vi "DataSync.vi"(8 "method":i32(ring)=1 caption="메소드" items=["최근접", "선형", "스플라인", "3차 에르미트", "라그랑지"], 9 "samples":i32=3000 caption="샘플", 10 "Y":dbl[](array[numeric]) format="%_6g", 11 "X":dbl[](array[numeric]) format="%_6g") -> (1 "yi":dbl[](array[numeric]) format="%_6g", 2 "xi used":dbl[](array[numeric]) caption="사용된 xi" format="%_6g", 3 "출력 웨이브폼":waveform(dbl))   [LabVIEW 2013]
uses:
  <vilib>/Analysis/1siggen.llb/Ramp Pattern by Samples.vi
  <vilib>/Analysis/NI_AALBase.lvlib
  <vilib>/gmath/NI_Gmath.lvlib
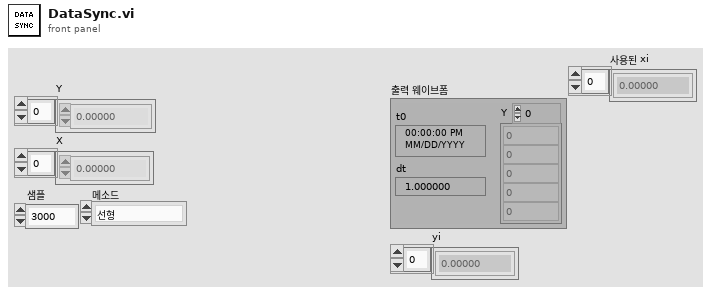
[diagram p1: front panel]
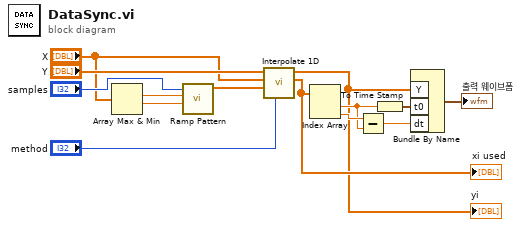
[diagram p0: block diagram]
diagram:
  n1 = Array Max & Min(array="X") -> (max value=w7:dbl, min value=w6:dbl)  [unwired: 2 out]
  n2 = call-poly <vilib>:"Ramp Pattern.vi"("start"=w6, "end"=w7, "samples"="samples") -> ("Ramp Pattern"=w14:dbl[])  [unwired: 7 in, 1 out]
  n3 = call <vilib>:"Interpolate 1D.vi"("method"="method", "xi"=w14, "X"="X", "Y"="Y") -> ("xi used"=w13:dbl[], "yi"=w8:dbl[])  [unwired: 5 in, 1 out]
  "yi" <- w8
  "xi used" <- w13
  n4 = Index Array(array=w13) -> (element #1=w10:dbl, element #2=w11:dbl)  [unwired: 2 in]
  n5 = Subtract(x=w11, y=w10) -> (x-y=w9:dbl)
  n6 = To Time Stamp(1:w10) -> (0:w12:timestamp)
  n7 = Bundle By Name("Y"=w8, "t0"=w12, "dt"=w9) -> (→"출력 웨이브폼":waveform(dbl))  [unwired: 1 in]
